vi "FPGA Input Write.vi"(8 "error in (no error)":errorcluster, 11 "RT data in":T1) -> (0 "error out":errorcluster, 3 "RT data out":T1)   [LabVIEW 2011, in "Engine Sim RT.lvlib"]
uses:
  Engine Sim RT.lvlib
  TypeDefs/RT Data Cluster.ctl
  Shared/Channel Descriptors.ctl
  Shared/FPGA Write Descriptor.ctl
  Shared/InputChannelTypes.ctl
  <vilib>/rvi/DataTransferAndStorage/Container/Common/niFpgaDataTypeControl.ctl
  Shared/FPGA Read Descriptor.ctl
  Shared/OutputChannelTypes.ctl
  Shared/Status Chan Descriptor.ctl
  Shared/DataReplayVoltageConfig.ctl
  <userlib>/_FPGA Interface Advanced Tools/FPGA Interface Wrapper/NiFPGA Write - U64.vi
  <vilib>/Utility/error.llb/Error Cluster From Error Code.vi
  <userlib>/_FPGA Interface Advanced Tools/FPGA Interface Wrapper/FPGA Interface Wrapper.lvlib
  Engine Simulation Shared.lvlib
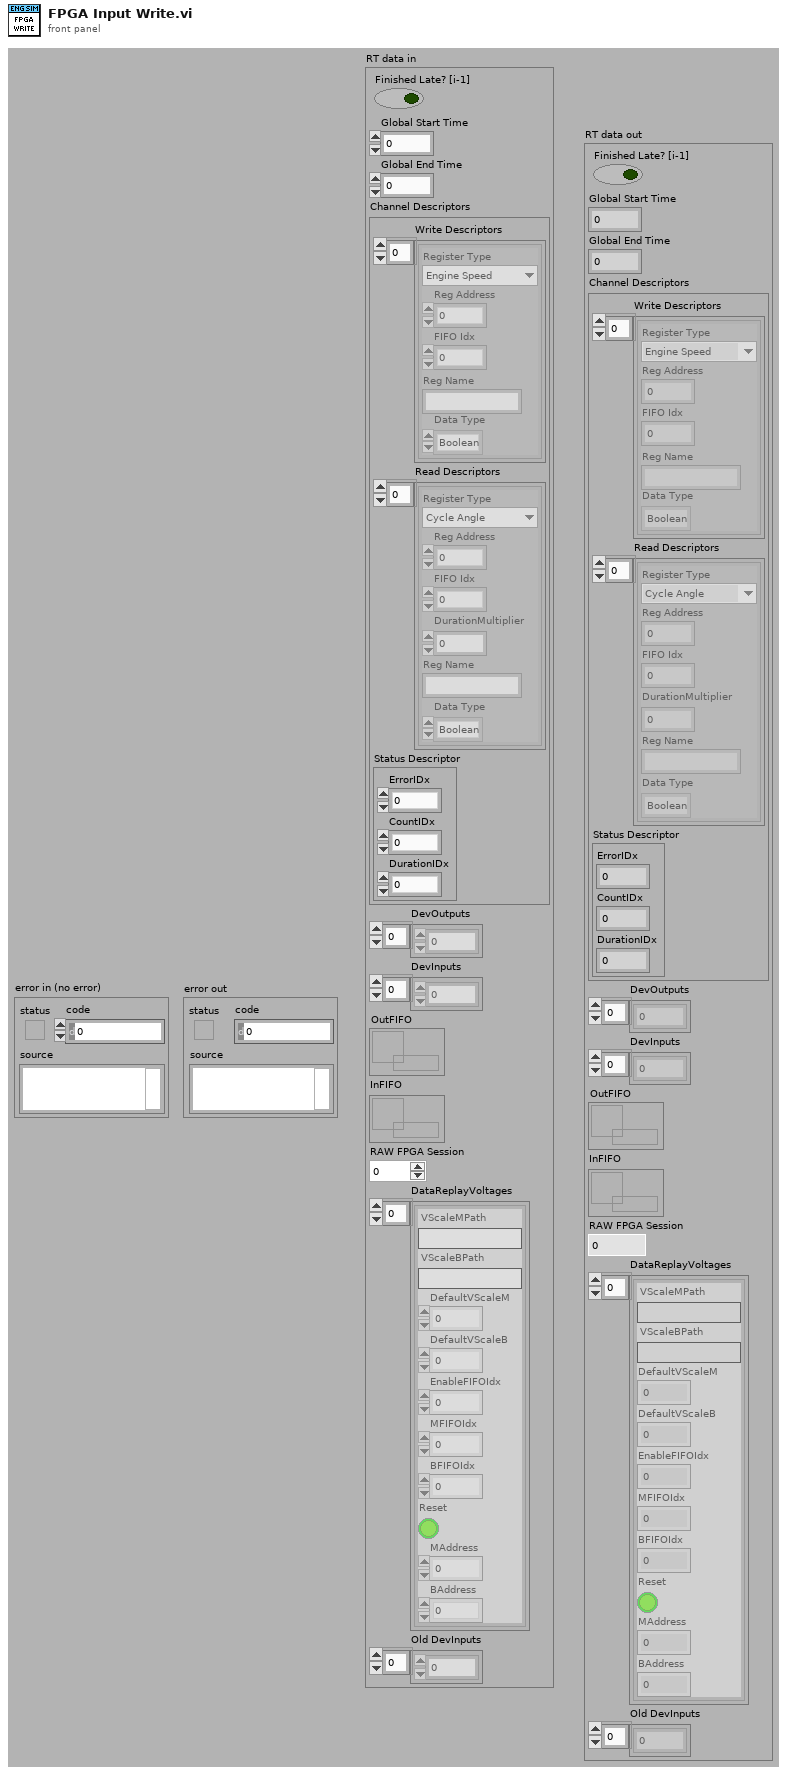
[diagram p1: front panel]
types:
  T1 = typedef "Engine Sim RT.lvlib/RT Data Cluster.ctl" = cluster{"Finished Late? [i-1]":bool, "Global Start Time":i64, "Global End Time":i64, "Channel Descriptors":T2, "DevOutputs":dbl[], "DevInputs":dbl[], "OutFIFO":refnum<k33>, "InFIFO":refnum<k33>, "RAW FPGA Session":u32, "DataReplayVoltages":T9[], "Old DevInputs":dbl[]}
  T2 = typedef "Engine Simulation Shared.lvlib/Channel Descriptors.ctl" = cluster{"Write Descriptors":T3[], "Read Descriptors":T6[], "Status Descriptor":T8}
  T3 = typedef "Engine Simulation Shared.lvlib/FPGA Write Descriptor.ctl" = cluster{"Register Type":T4, "Reg Address":u32, "FIFO Idx":i32, "Reg Name":string, "Data Type":T5}
  T4 = typedef "Engine Simulation Shared.lvlib/InputChannelTypes.ctl" = enum16{"Engine Speed", "Offset"}
  T5 = typedef "niFpgaDataTypeControl.ctl" = enum32{"Boolean", "I8", "I16", "I32", "I64", "U8", "U16", "U32", "U64", "FXP", "CustomControl"}
  T6 = typedef "Engine Simulation Shared.lvlib/FPGA Read Descriptor.ctl" = cluster{"Register Type":T7, "Reg Address":u32, "FIFO Idx":i32, "DurationMultiplier":dbl, "Reg Name":string, "Data Type":T5}
  T7 = typedef "Engine Simulation Shared.lvlib/OutputChannelTypes.ctl" = enum16{"Cycle Angle", "Crank Angle", "Time Duration", "Angle Duration", "Start Angle", "End Angle"}
  T8 = typedef "Engine Simulation Shared.lvlib/Status Chan Descriptor.ctl" = cluster{"ErrorIDx":i32, "CountIDx":i32, "DurationIDx":i32}
  T9 = typedef "Engine Simulation Shared.lvlib/DataReplayVoltageConfig.ctl" = cluster{"VScaleMPath":string, "VScaleBPath":string, "DefaultVScaleM":u32, "DefaultVScaleB":i32, "EnableFIFOIdx":i32, "MFIFOIdx":i32, "BFIFOIdx":i32, "Reset":bool, "MAddress":u32, "BAddress":u32}
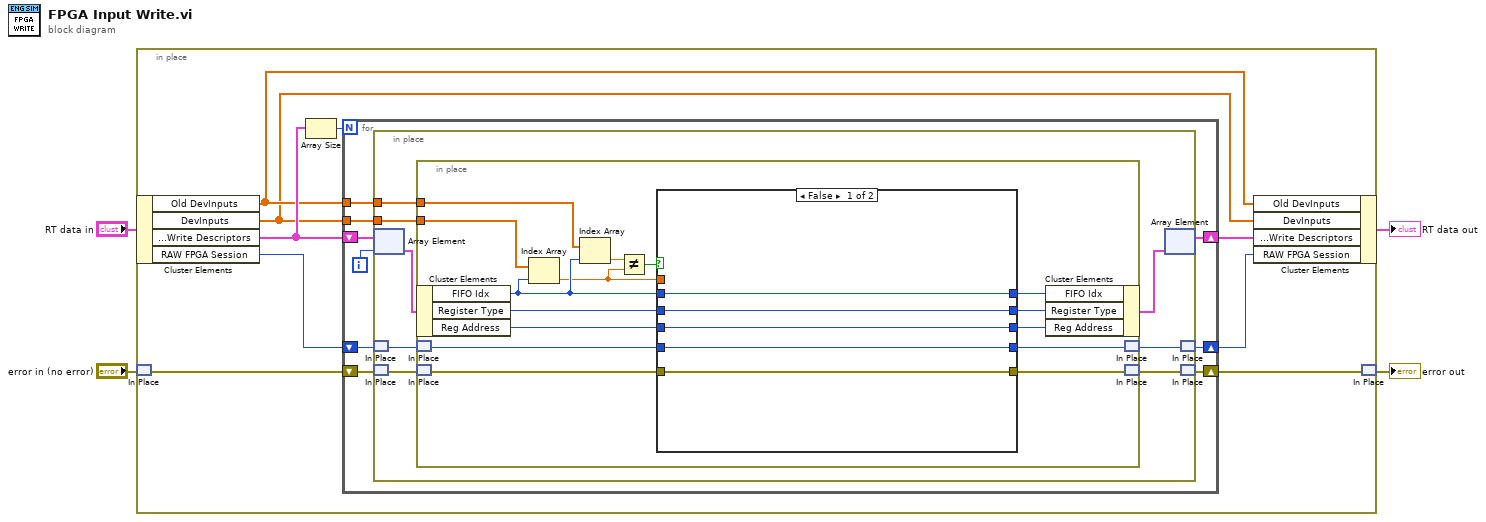
[diagram p0: block diagram]
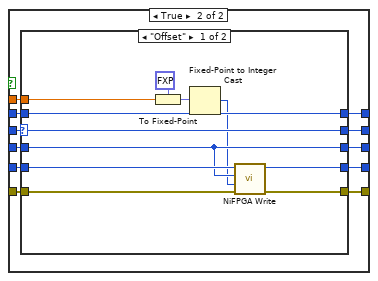
[diagram p2: hidden frame]
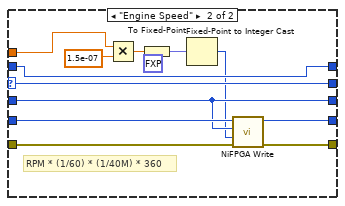
[diagram p3: hidden frame]
diagram:
  n1 = in-place {
    n2 = in-place-cluster #1("RT data in") -> ("Old DevInputs"=w6:dbl[], "DevInputs"=w5:dbl[], "Channel Descriptors.Write Descriptors"=w11:T3[], "RAW FPGA Session"=w10:u32)
    n3 = in-place-match #2("error in (no error)") -> (w8:errorcluster)
    n4 = Array Size(array=w11) -> (size(s)=w12:i32)
    n5 = for {
      N: w12 -> [_]
      shift-right: [w22] -> w7
      shift-left: w8 -> [w21]
      shift-right: [w19] -> w13
      shift-left: w11 -> [w20]
      shift-right: [w17] -> w9
      shift-left: w10 -> [w18]
      tunnel: w5 -> [w15]
      tunnel: w6 -> [w14]
      i -> [w16]
      n6 = in-place {
        in-place-border: w15 -> [w24]
        in-place-border: w14 -> [w23]
        n7 = in-place-array #3(w20, w16) -> (w28:T3)
        n8 = in-place-match #4(w18) -> (w26:u32)
        n9 = in-place-match #5(w21) -> (w29:errorcluster)
        n10 = in-place {
          in-place-border: w24 -> [w33]
          in-place-border: w23 -> [w32]
          n11 = in-place-cluster #6(w28) -> ("FIFO Idx"=w36:i32, "Register Type"=w40:T4, "Reg Address"=w41:u32)
          n12 = in-place-match #7(w26) -> (w43:u32)
          n13 = in-place-match #8(w29) -> (w45:errorcluster)
          n14 = Index Array(array=w33, index=w36) -> (element=w34:dbl)
          n15 = Index Array(array=w32, index=w36) -> (element=w35:dbl)
          n16 = Not Equal?(x=w35, y=w34) -> (x != y?=w31:bool)
          n17 = case shown="False" w31 {
            tunnel: w45 -> [w46 w61]
            tunnel: [w46 w60] -> w44
            tunnel: w43 -> [w47 w59]
            tunnel: [w47 w58] -> w42
            tunnel: w41 -> [w48 w57]
            tunnel: w40 -> [w49 w56]
            tunnel: [w50 w55] -> w39
            tunnel: [w49 w54] -> w38
            tunnel: [w48 w53] -> w37
            tunnel: w36 -> [w50 w52]
            tunnel: w34 -> [_ w51]
            frame False {
            }
            frame True {
              n18 = case shown="\"Offset\"" w56 {
                selector: w56 -> [w67 w80]
                tunnel: w57 -> [w68 w81]
                tunnel: w61 -> [w72 w85]
                tunnel: [w71 w84] -> w60
                tunnel: w59 -> [w70 w83]
                tunnel: [w69 w82] -> w58
                tunnel: w52 -> [w66 w79]
                tunnel: [w66 w79] -> w55
                tunnel: [w67 w80] -> w54
                tunnel: [w68 w81] -> w53
                tunnel: w51 -> [w65 w78]
                frame "Offset" {
                  n19 = To Fixed-Point(fixed-point type=fxp<+/-,61,10> 0.0 ("FullyCustomTeeth.Cams.Cam1.Offset"), number=w65) -> (fixed-point=w63:fxp<+/-,61,10>)
                  n20 = Fixed-Point to Integer Cast(1:w63) -> (0:w62:i64)
                  n21 = call-poly <userlib>:"NiFPGA Write.vi"("error in (no error)"=w72, "Value"=w62, "Control"=w68, "Session"=w70) -> ("error out"=w71:errorcluster, "Session Out"=w69:u32)  [unwired: 6 in]
                }
                frame "Engine Speed" {
                  # "RPM * (1/60) * (1/40M) * 360"
                  n22 = Multiply(x=w78, y=1.5e-07) -> (x*y=w75:dbl)
                  n23 = To Fixed-Point(fixed-point type=fxp<+/-,47,-4> 0.0 ("Degrees/Tooth"), number=w75) -> (fixed-point=w73:fxp<+/-,47,-4>)
                  n24 = Fixed-Point to Integer Cast(1:w73) -> (0:w77:i64)
                  n25 = call-poly <userlib>:"NiFPGA Write.vi"("error in (no error)"=w85, "Value"=w77, "Control"=w81, "Session"=w83) -> ("error out"=w84:errorcluster, "Session Out"=w82:u32)  [unwired: 6 in]
                }
              }
            }
          }
          n26 = in-place-cluster #6("FIFO Idx"=w39, "Register Type"=w38, "Reg Address"=w37) -> (w27:T3)
          n27 = in-place-match #7(w42) -> (w25:u32)
          n28 = in-place-match #8(w44) -> (w30:errorcluster)
        }
        n29 = in-place-array #3(w27) -> (w19:T3[])  [unwired: 1 out]
        n30 = in-place-match #4(w25) -> (w17:u32)
        n31 = in-place-match #5(w30) -> (w22:errorcluster)
      }
    }
    n32 = in-place-cluster #1("Old DevInputs"=w6, "DevInputs"=w5, "Channel Descriptors.Write Descriptors"=w13, "RAW FPGA Session"=w9) -> (→"RT data out":T1)
    n33 = in-place-match #2(w7) -> (→"error out":errorcluster)
  }
